vi "Get_Status_of_Displacement-1.vi"(4 "[IN] Dot matrix with statuses\nfor potentially moving dots":i16[][](array[numeric]), 6 "[IN] Potentially\nMoving (X,Y)":dbl[][](array[numeric]), 7 "[IN] Start pos":i32, 8 "[IN] Index of Problem\nPoint in Subtrack":i32, 9 "[IN] Subtrack":dbl[](array[numeric]), 10 "[IN] Index of\n subtrack":i32, 11 "[IN] Displace-\nment Statuses":i16[](array[numeric])) -> (3 "[OUT] Displace\nment Statuses":i16[](array[numeric]))   [LabVIEW 2017]
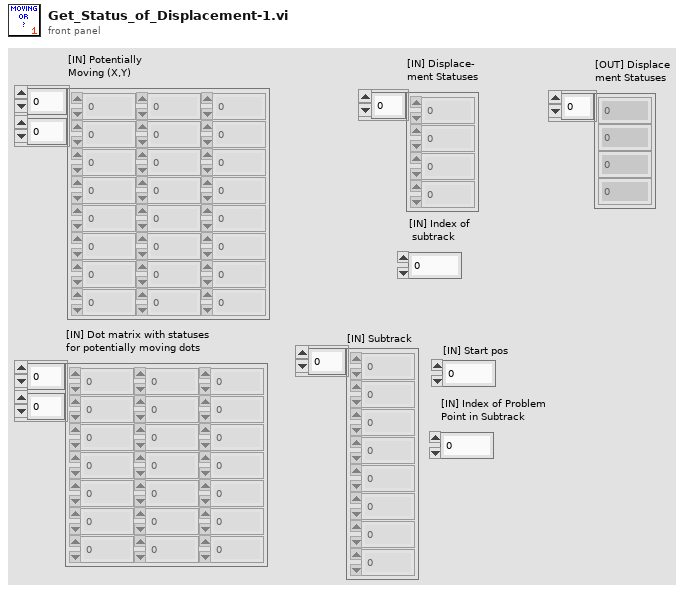
[diagram p1: front panel]
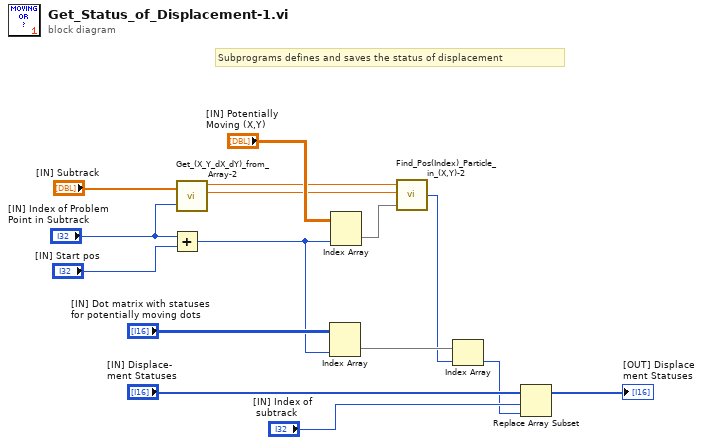
[diagram p0: block diagram]
diagram:
  # "Subprograms defines and saves the status of displacement"
  n1 = Add(x="[IN] Index of Problem\nPoint in Subtrack", y="[IN] Start pos") -> (x+y=w9:i32)
  n2 = call "Get_(X_Y_dX_dY)_from_Array-2.vi"("(X,Y,dX,dY)"="[IN] Subtrack", "Index of Displacement"="[IN] Index of Problem\nPoint in Subtrack") -> ("X"=w2:dbl, "Y"=w1:dbl)  [unwired: 2 out]
  n3 = Index Array(array="[IN] Dot matrix with statuses\nfor potentially moving dots", index (col)=w9) -> (element=w8:i16[])  [unwired: 1 in]
  n4 = Index Array(array="[IN] Potentially\nMoving (X,Y)", index (col)=w9) -> (element=w11:dbl[])  [unwired: 1 in]
  n5 = call "Find_Pos(Index)_Particle_in_(X,Y)-2.vi"("[X,Y] (n Frame)"=w11, "Y1"=w1, "X1"=w2) -> ("Index in (n) Frame"=w7:i32)
  n6 = Index Array(array=w8, index=w7) -> (element=w4:i16)
  n7 = Replace Array Subset(array="[IN] Displace-\nment Statuses", new element=w4, index="[IN] Index of\n subtrack") -> (→"[OUT] Displace\nment Statuses":i16[])
